vi "Intake_Joint_Globals.vi"() -> ()   [LabVIEW 2018]
uses:
  Subsytems/Intake_Joint/Intake_Joint_Notifier.ctl
  Subsytems/Intake_Joint/Intake_Joint_Control_Type.ctl
panel:
  in  "Bottom_Joint_Limit":string="Bottom_Joint_Limit"
  in  "Top_Joint_Limit":string="Top_Joint_Limit"
  in  "Intake_Joint_Set_Ref":refnum<notifier>
  in  "Intake_Joint_Execution_Ref":refnum<notifier>
  in  "Intake_Joint_Execute_Notifier":string="Intake_Joint_Execute_Notifier"
  in  "Intake_Joint_Set_Notifier":string="Intake_Joint_Set_Notifier"
  in  "Joint_Motor":string="Joint_Motor"
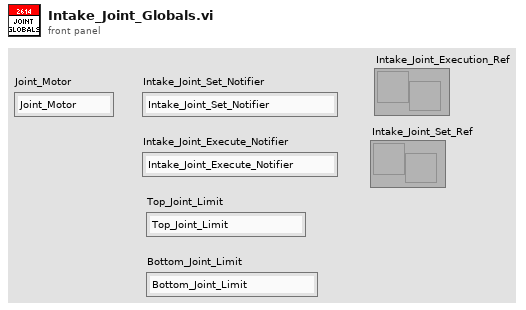
[diagram p1: front panel]
diagram:
